vi "Update APU Name.vi"(8 "error in (no error)":errorcluster, 11 "APU Select":T1="<Select>") -> (0 "error out":errorcluster)   [LabVIEW 2018]
doc: "This subVI enqueues the named action in to the communications queue along with the input data."
uses:
  Private Controls/Module Action.ctl
  Controller (Host)/Public Controls/APU Select.ctl
  Private Controls/Module Data.ctl
  Testing UI 1.lvlib
  Controller (Host)/Controller (Host).lvlib
panel:
  in  "Action":T2=enum."Update APU Name"
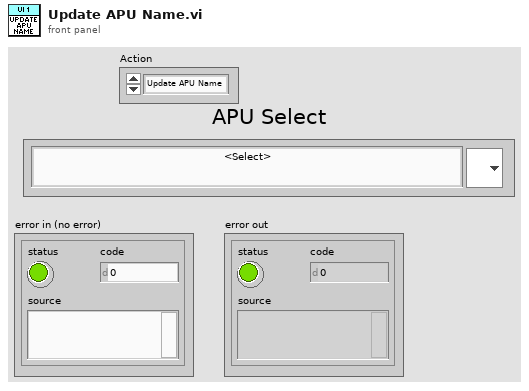
[diagram p1: front panel]
types:
  T1 = typedef "Controller (Host).lvlib/APU Select.ctl" = string
  T2 = typedef "Testing UI 1.lvlib/Module Action.ctl" = enum8{"Timeout", "Init", "Error", "Exit", "HideShow FP", "Send Control Vals", "New Message Line", "Update System Log", "Load APU Setup Data", "Update APU Name", "Set Testing Type", "Threshold ALERT", "Set Rapid OpenORClose", "Engine Start Val Change", "Fault Trip Run Updater", " ---------------UI 4 APIs ---------------", "UI 4 Engine Start Val Change", "UI 4 Fuel Pressure Reg Val Change", "U1 4 APU & ECU Control Val Change", "UI 4 Bleed Load Val Change", "UI4 Testing Controls Val Change", "UI4 Break Out Val Change", "UI4 Crash Log Val Change", "UI4 Log Data Val Change", "UI4 Sampes-Sec Val Change", "Update Run Count", "Config Interactive Ctrls"}
  T3 = typedef "Testing UI 1.lvlib/Module Data.ctl" = cluster{"Data":variant, "Action":T2}
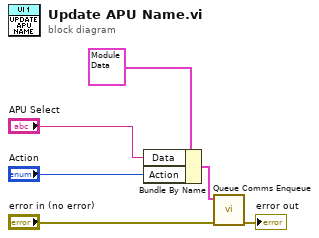
[diagram p0: block diagram]
diagram:
  n1 = Bundle By Name(cluster=T3 {"Data"=variant, "Action"=enum."Init"} ("element"), "Data"="APU Select", "Action"="Action") -> (w6:T3)
  n2 = call "Queue Comms Enqueue.vi"("error in (no error)"="error in (no error)", "element"=w6) -> ("error out"=→"error out":errorcluster)  [unwired: 9 in]
